vi "Fold Windowed Signal.vi"(10 "frequency bins":i32, 11 "Windowed Signal":dbl[](array[numeric])) -> (3 "Folded Signal":dbl[](array[numeric]))   [LabVIEW 2017, in "NI_Gmath.lvlib"]
uses:
  NI_Gmath.lvlib
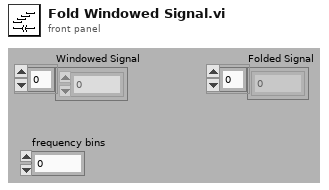
[diagram p1: front panel]
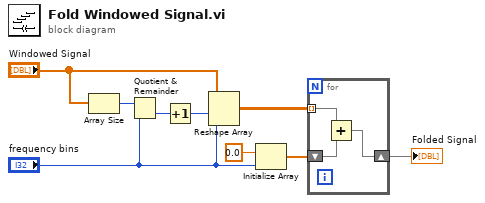
[diagram p0: block diagram]
diagram:
  n1 = Array Size(array="Windowed Signal") -> (size(s)=w2:i32)
  n2 = Quotient & Remainder(x=w2, y="frequency bins") -> (floor(x/y)=w3:i32)  [unwired: 1 out]
  n3 = Increment(x=w3) -> (x+1=w4:i32)
  n4 = Reshape Array("Windowed Signal", w4, "frequency bins") -> (w7:dbl[][])
  n5 = Initialize Array(0.0 ("element"), "frequency bins") -> (w6:dbl[])
  n6 = for {
    shift-right: [w10] -> w8
    shift-left: w6 -> [w11]
    tunnel: w7 -> [w12] mode=indexing
    n7 = Add(x=w12, y=w11) -> (x+y=w10:dbl[])
  }
  "Folded Signal" <- w8
